vi "WAV_Master.vi"() -> ()   [LabVIEW 2022 SP3]
uses:
  PreferencesControl.ctl
  <vilib>/Utility/miscctls.llb/LVSelectionTypeDef.ctl
  <vilib>/Utility/error.llb/Trim Whitespace One-Sided.vi
panel:
  out "names":string[](array[string])
  out "wfm":waveform(dbl)[](graph)
  in  "Tab Control":enum32{"Intro", "Params", "Settings", "Saving"}(tab)
  out "Number of taps":i32
  out "raw file":string
  in  "Set Name":string="H"
  in  "Tap number":u32=1
  in  "Position":u32=1
  in  "Settings":T1={"Name of test"="name", "Date"=timestamp(0 s since 1904-01-01), "Location"="Home", "Template"="wav translator", "Soundcard"="OCTA-CAPTURE", "resolution"=32, "Sampling rate"=48000, "Ch1 Gain "=10.0, "Ch2 Gain"=20.0, "Sample time (s)"=0.3, "Pre-trigger (s)"=0.001, "Hammer Threshold"=0.01, "Positions"=12, "Taps/Position"=5, "Set Names"="H,V", "Freq resolution"=1.0, "Hammer cutoff"=0.025, "Mic cutoff"=0.25, "Double bounce "=0.01, "Hammer Cal"=23.6, "dB Offset"=0.0, "Accel Cal"=1.014, "Vibrometer Cal"=1.0, "Mic Cal"=48.5, "Output"=2, "Voltage Cal"=3.8, "Vibrometer Port"="ASRL27::INSTR", "Range"=50, "High Pass"=2, "Bandwidth"=25, "X Range"=[{"Minimum"=200.0, "Maximum"=10000.0, "Increment"=2500.0, "Minor Increment"=500.0, "Start"=2500.0}, {"Minimum"=0.0, "Maximum"=0.05, "Increment"=0.025, "Minor Increment"=0.0025, "Start"=0.0}, {"Minimum"=0.0, "Maximum"=0.3, "Increment"=0.1, "Minor Increment"=0.01, "Start"=0.0}, {"Minimum"=200.0, "Maximum"=10000.0, "Increment"=10.0, "Minor Increment"=100.0, "Start"=1000.0}], "Y Range"=[{"Minimum"=-25.0, "Maximum"=0.0, "Increment"=5.0, "Minor Increment"=1.0, "Start"=-25.0}, {"Minimum"=-0.1, "Maximum"=1.0, "Increment"=0.25, "Minor Increment"=0.05, "Start"=0.0}, {"Minimum"=-1.0, "Maximum"=1.0, "Increment"=0.5, "Minor Increment"=0.1, "Start"=-1.0}, {"Minimum"=-10.0, "Maximum"=30.0, "Increment"=10.0, "Minor Increment"=0.5, "Start"=-10.0}], "dB Spread"=40.0, "Trigger"=0, "Ch_1"=2, "Ch_2"=1, "flip?"=FALSE, "60Hz"=FALSE, "Time offset"=0.0, "Piezo Cal"=1.0, "Default Notes"=""} {"Ch_2" min=1 step=1; "Ch_1" min=1 max=100 step=1; "Trigger" items=["Hammer (force)", "Self-tap", "Spacebar"]; "Bandwidth" items=["1 kHz"=1, "5 kHz"=5, "10 kHz"=10, "25 kHz"=25, "50 kHz"=50, "100 kHz"=100]; "High Pass" items=["Off", "13 Hz", "104 Hz"]; "Range" items=["10 mm/s"=1, "20 mm/s"=2, "50 mm/s"=5, "100 mm/s"=10, "200 mm/s"=20, "500 mm/s"=50, "1 m/s"=100, "2 m/s"=200]; "Output" items=["Accelerometer", "Speed (from acceleration)", "Microphone", "Vibrometer", "Piezo"]; "Voltage Cal" format="%#_13g"; "Ch2 Gain" format="%#_13g"; "Ch1 Gain" format="%#_13g"; "Double bounce" min=0.0; "Mic cutoff" min=0.0 format="%#_4g"; "Hammer cutoff" min=0.0 format="%#_4g"; "Freq resolution" min=0.0; "Pre-trigger (s)" format="%#_13g"; "Date" format="%<%H:%M\n%d/%m/%y>T"; "resolution" items=["16 bit"=16, "24 bit"=24, "32 bit"=32]; "Sampling rate" items=["22050 samp/s"=22050, "44100 samp/s"=44100, "48000 samp/s"=48000]}
  in  "Test Name":string
  in  "Files":i32(listbox)=-1
  in  "Save Button":bool
  in  "Instrument Name":string(combo)
  in  "View Settings":bool
  in  "wav folder path":path
  out "FRF":cluster{"x0":dbl, "df":dbl, dbl[]}(graph)
  in  "play selection":bool
  out "File name":string
  out "data":T2={"Hammer"=[], "Hammer Spectra"=[{1.0, "df"=1.0, "FFT {X}"=array[24000 elements]}], "Microphone"=[{0.0, "dt"=2.0833333333333333e-05, "Y"=array[14400 elements]}], "Microphone Spectra"=[{"x0"=1.0, "df"=1.0, array[24000 elements]}], "Average FRF"=[{1.0, "df"=1.0, array[24000 elements]}, {1.0, "df"=1.0, array[24000 elements]}]}
  in  "Back":bool
  out "Slide":u8(slide) scale=0.0..100.0
  # "Welcome To The WAV File Translator"
  # "This will translate a wav file and let you play it"
  # "1. Select a folder of wav files\nHit the folder button or drag a file on"
  # "2. Define an instrument and settings\nAdd to an existing or create a new instrument\nand edit settings (or use defaults)"
  # "3. Translate the data\nMake sure the data looks good"
  # "4. Specify start Set, position, and hit\nall gets added to the data file name"
  # "5. Repeat or Close\nSelect a new file or close the window"
  # "Hz"
  # "dB"
  # "dB"
  # "sec"
  # "sec"
  # "mV/Pa"
  # "mV/m/s2"
  # "mV/mm/s"
  # "V/N"
  # "sec"
  # "sec"
  # "mV/N"
  # "a.u."
  # "a.u."
  # "sec"
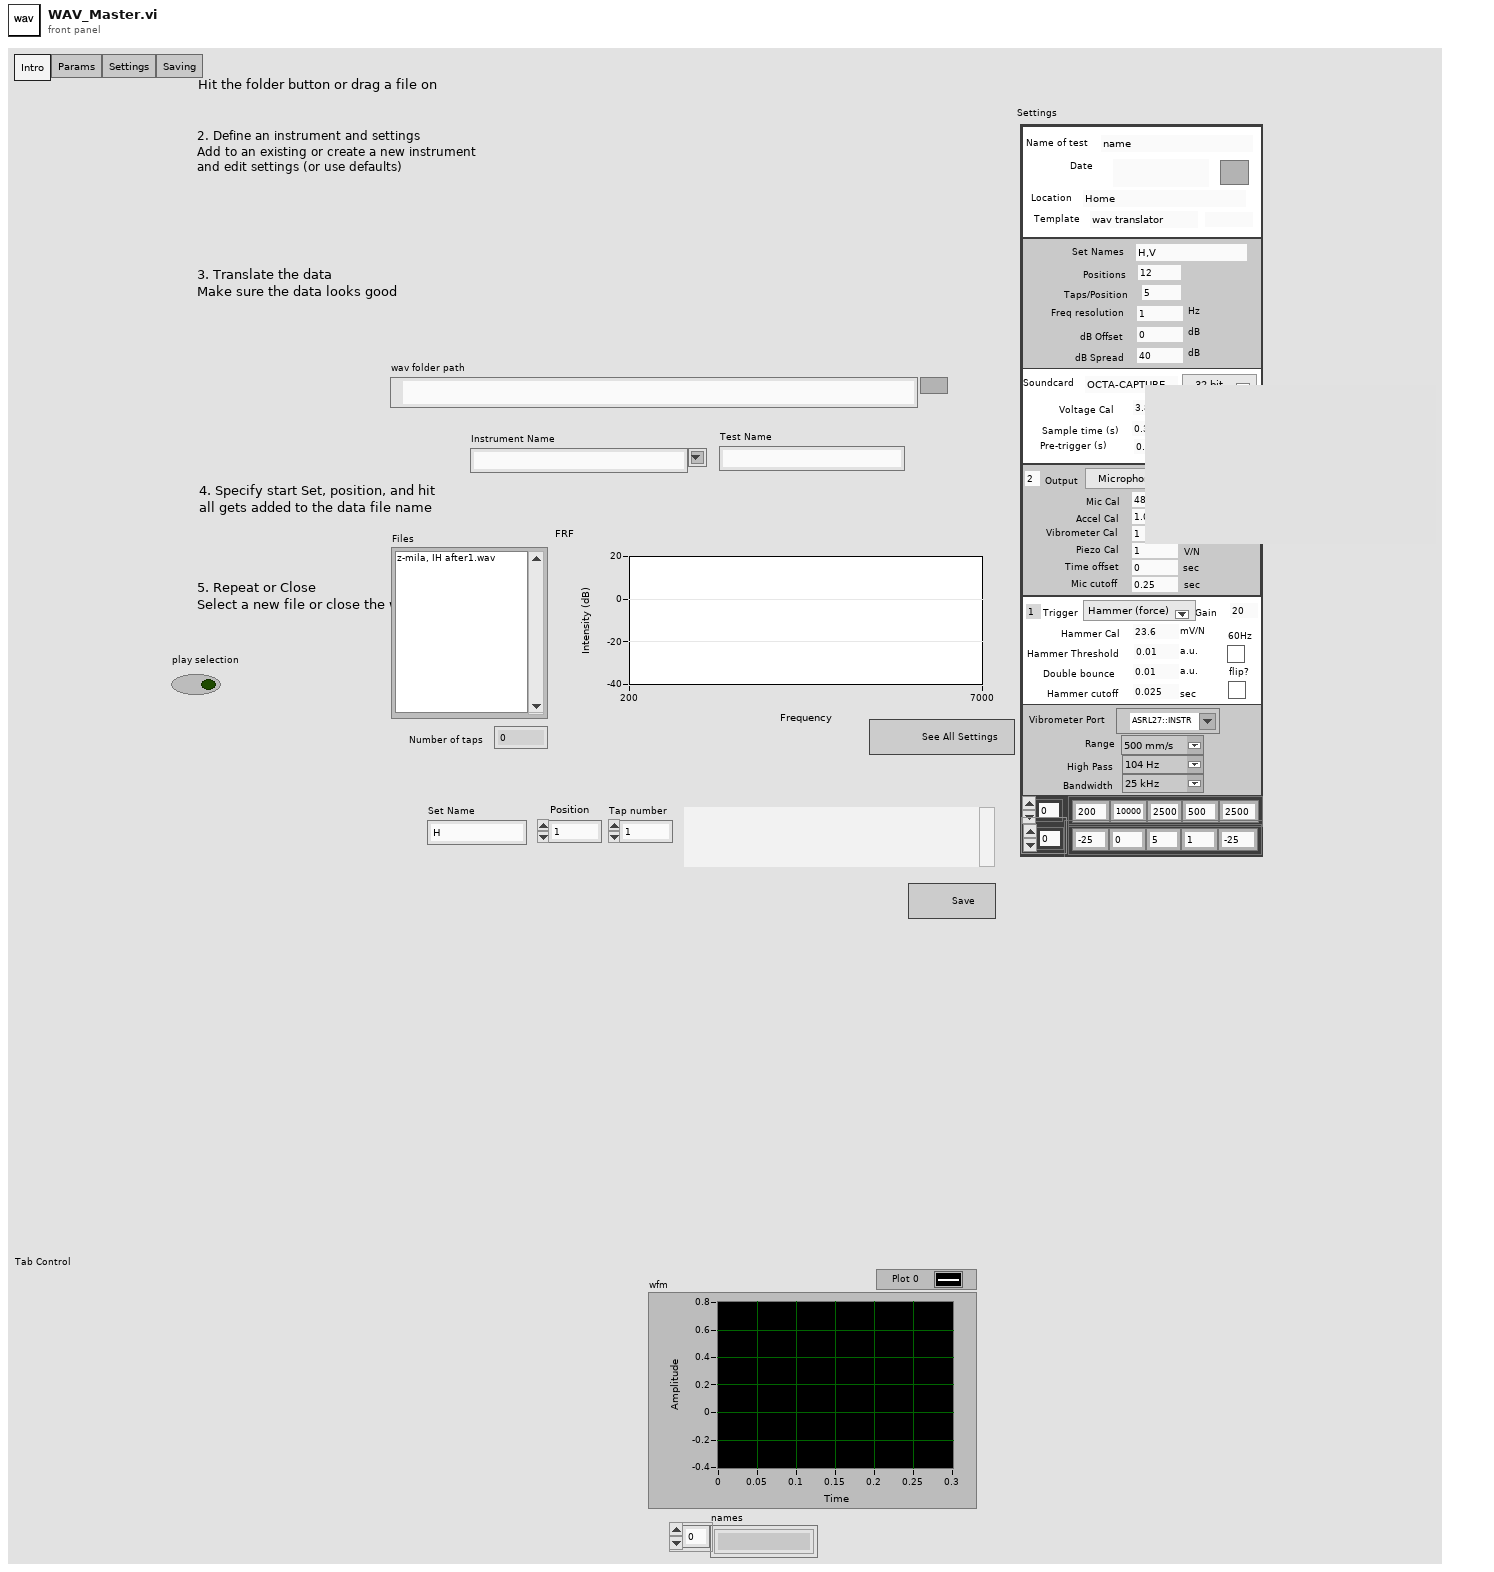
[diagram p1: front panel]
types:
  T1 = typedef "PreferencesControl.ctl" = cluster{"Name of test":string, "Date":timestamp, "Location":string, "Template":string, "Soundcard":string, "resolution":u16, "Sampling rate":u16, "Ch1 Gain ":dbl, "Ch2 Gain":dbl, "Sample time (s)":dbl, "Pre-trigger (s)":dbl, "Hammer Threshold":dbl, "Positions":i16, "Taps/Position":i16, "Set Names":string, "Freq resolution":dbl, "Hammer cutoff":dbl, "Mic cutoff":dbl, "Double bounce ":dbl, "Hammer Cal":dbl, "dB Offset":dbl, "Accel Cal":dbl, "Vibrometer Cal":dbl, "Mic Cal":dbl, "Output":u16, "Voltage Cal":dbl, "Vibrometer Port":refnum<visa-resource-name>, "Range":u16, "High Pass":u16, "Bandwidth":u16, "X Range":cluster{"Minimum":dbl, "Maximum":dbl, "Increment":dbl, "Minor Increment":dbl, "Start":dbl}[], "Y Range":cluster{"Minimum":dbl, "Maximum":dbl, "Increment":dbl, "Minor Increment":dbl, "Start":dbl}[], "dB Spread":dbl, "Trigger":u16, "Ch_1":u8, "Ch_2":u8, "flip?":bool, "60Hz":bool, "Time offset":dbl, "Piezo Cal":dbl, "Default Notes":string}
  T2 = cluster{"Hammer":cluster{dbl, "dt":dbl, "Y":dbl[]}[], "Hammer Spectra":cluster{dbl, "df":dbl, "FFT {X}":dbl[]}[], "Microphone":cluster{dbl, "dt":dbl, "Y":dbl[]}[], "Microphone Spectra":cluster{"x0":dbl, "df":dbl, dbl[]}[], "Average FRF":cluster{dbl, "df":dbl, dbl[]}[]}
  T3 = enum8{"Enabled", "Disabled", "Disabled and Grayed Out"}
  T4 = typedef "LVSelectionTypeDef.ctl" = cluster{"Selection Start":u32, "Selection End":u32}
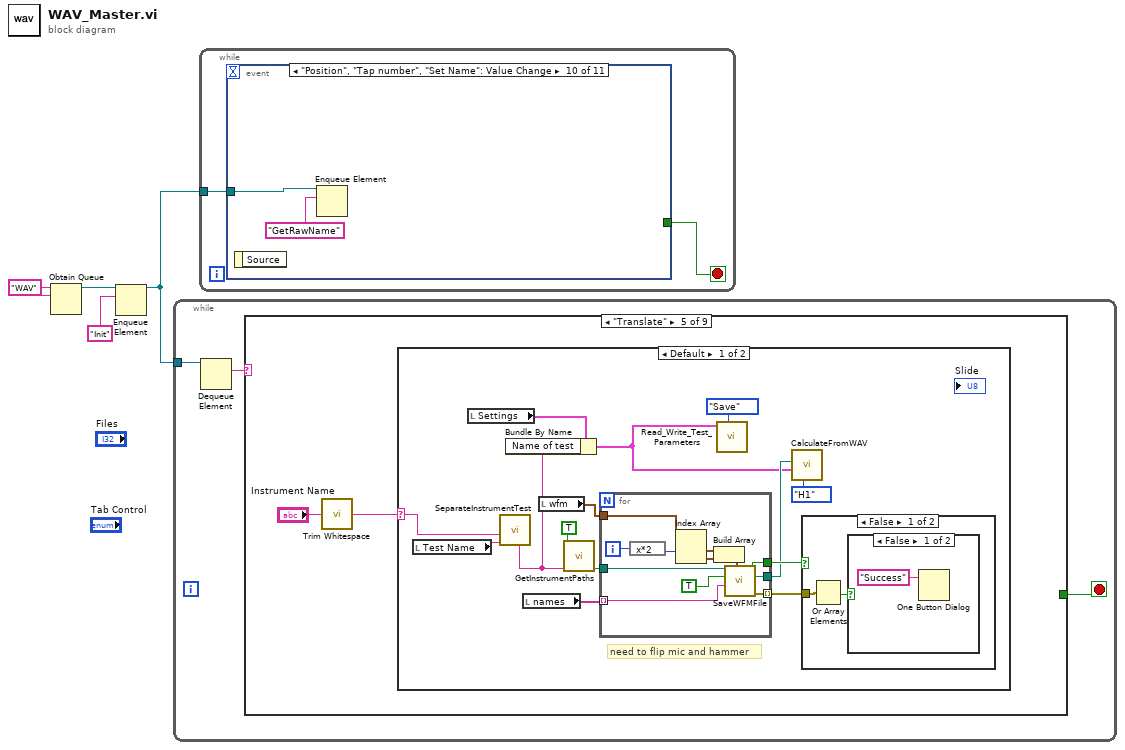
[diagram p0: block diagram]
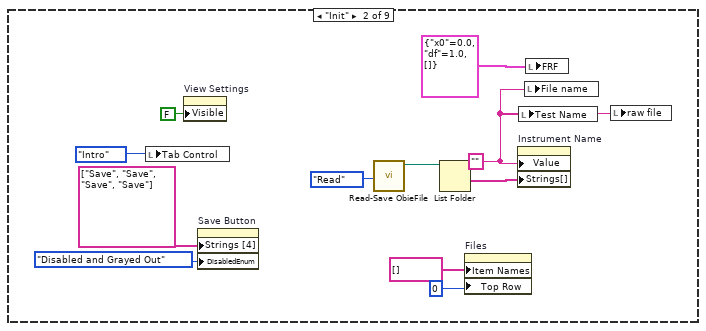
[diagram p3: hidden frame]
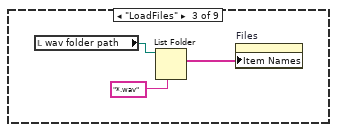
[diagram p4: hidden frame]
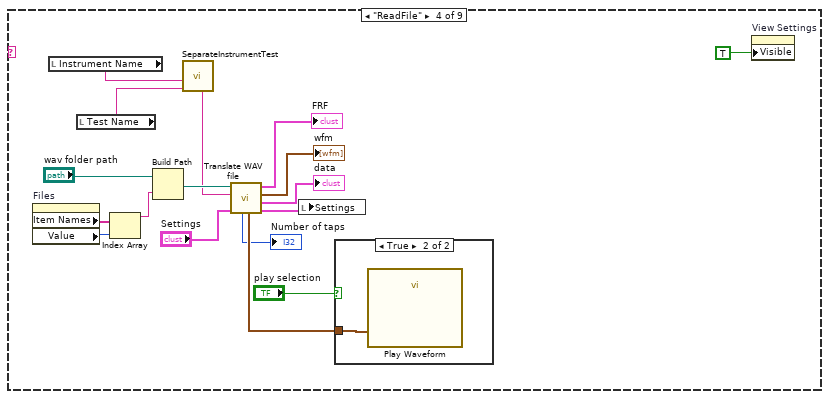
[diagram p5: hidden frame]
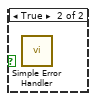
[diagram p7: hidden frame]
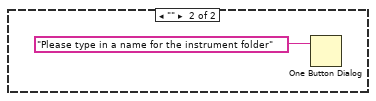
[diagram p9: hidden frame]
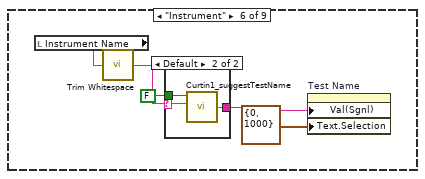
[diagram p10: hidden frame]
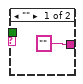
[diagram p11: hidden frame]
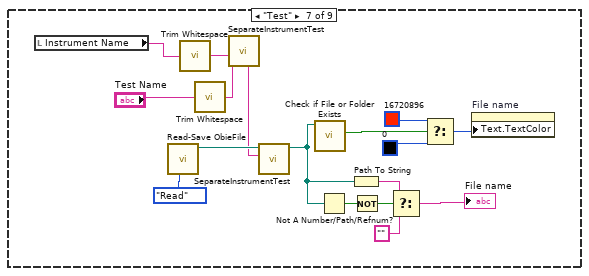
[diagram p12: hidden frame]
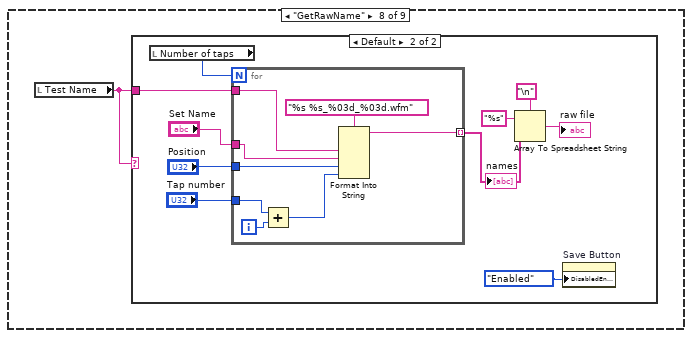
[diagram p13: hidden frame]
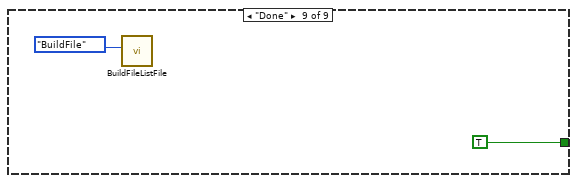
[diagram p15: hidden frame]
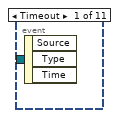
[diagram p16: hidden frame]
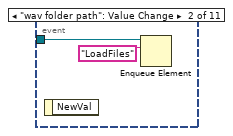
[diagram p17: hidden frame]
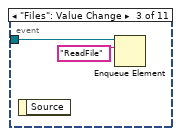
[diagram p18: hidden frame]
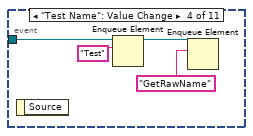
[diagram p19: hidden frame]
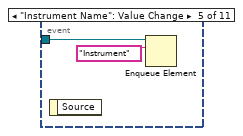
[diagram p20: hidden frame]
diagram:
  w4 = "WAV" ("name (unnamed)")
  n1 = Obtain Queue(name (unnamed)=w4, element data type=w4) -> (queue out=w2:refnum<queue>)  [unwired: 3 in, 2 out]
  n2 = Enqueue Element(queue=w2, element="Init") -> (queue out=w1:refnum<queue>)  [unwired: 2 in, 2 out]
  n3 = while {
    tunnel: w1 -> [w7]
    stop <- w5 stop-if-true
    n4 = Dequeue Element(queue=w7) -> (element=w6:string)  [unwired: 2 in, 3 out]
    n5 = case shown="\"Translate\"" w6 {
      tunnel: [_ _ _ _ _ _ _ _ TRUE ("Discard?")] -> w5
      frame Default {
      }
      frame "Init" {
        w8 = "" ("Value (Signaling)")
        n6 = local write "Tab Control"(enum32{"Intro", "Params", "Settings"}."Intro" ("Tab Control")) -> ()
        n7 = property on="View Settings" class="Bool"("Visible"=FALSE) -> ()  [unwired: 2 in, 2 out]
        n8 = property on="Save Button" class="Bool"("Strings [4]"=string[] ["Save", "Save", "Save", "Save"], "DisabledEnum"=T3."Disabled and Grayed Out" ("Disabled")) -> ()  [unwired: 2 in, 2 out]
        n9 = call "Read-Save ObieFile.vi"("Task"=enum16{"Save", "Read"}."Read") -> ("DataPath Out"=w15:path)  [unwired: 8 in, 2 out]
        n10 = List Folder(path=w15) -> (folder names=w14:string[])  [unwired: 3 in, 3 out]
        n11 = property on="Files" class="LstBox (strict)"("Item Names"=string[] [], "Top Row"=0) -> ()  [unwired: 2 in, 2 out]
        n12 = property on="Instrument Name" class="CmbBox"("Value"=w8, "Strings[]"=w14) -> ()  [unwired: 2 in, 2 out]
        n13 = local write "Test Name"(w8) -> ()
        n14 = local write "File name"(w8) -> ()
        n15 = local write "FRF"(cluster{"x0":dbl, "df":dbl, dbl[]} {"x0"=0.0, "df"=1.0, []} ("FRF")) -> ()
        n16 = local write "raw file"(w8) -> ()
      }
      frame "LoadFiles" {
        n17 = local read "wav folder path"() -> (w21:path)
        n18 = List Folder(path=w21, pattern="*.wav") -> (filenames=w19:string[])  [unwired: 2 in, 3 out]
        n19 = property on="Files" class="LstBox (strict)"("Item Names"=w19) -> ()  [unwired: 2 in, 2 out]
      }
      frame "ReadFile" {
        n20 = property on="Files" class="LstBox (strict)"() -> ("Item Names"=w33:string[], "Value"=w34:i32)  [unwired: 2 in, 2 out]
        n21 = local read "Instrument Name"() -> (w24:string)
        n22 = local read "Test Name"() -> (w25:string)
        n23 = Index Array(array=w33, index=w34) -> (element=w32:string)
        n24 = Build Path(base path="wav folder path", name or relative path=w32) -> (appended path=w30:path)
        n25 = call "SeparateInstrumentTest.vi"("test in"=w25, "Instrument in"=w24) -> ("Instrument -- test out"=w23:string)  [unwired: 5 in, 4 out]
        n26 = call "Translate WAV file.vi"("Settings"="Settings", "Name of test"=w23, "appended path"=w30) -> ("Settings Out"=w28:T1, 1:"data"=→"data":T2, "data 2"=→"wfm":waveform(dbl)[], "Average FRF out"=→"FRF":cluster{"x0":dbl, "df":dbl, dbl[]}, 4:"data"=w35:waveform(dbl)[], "# pts"=→"Number of taps":i32)  [unwired: 2 in, 1 out]
        n27 = local write "Settings"(w28) -> ()
        n28 = case shown="True" "play selection" {
          tunnel: w35 -> [_ w39]
          frame False {
          }
          frame True {
            n29 = call "Play Waveform"("Data"=w39) -> ()  [unwired: 18 in, 1 out]
          }
        }
        n30 = property on="View Settings" class="Bool"("Visible"=TRUE) -> ()  [unwired: 2 in, 2 out]
      }
      frame "Translate" {
        n31 = call <vilib>:"Trim Whitespace.vi"("string"="Instrument Name") -> ("trimmed string"=w40:string)  [unwired: 1 in]
        n32 = case shown="Default" w40 {
          selector: w40 -> [w50 _]
          frame Default {
            # "need to flip mic and hammer"
            n33 = local read "Test Name"() -> (w54:string)
            n34 = local read "Settings"() -> (w43:T1)
            n35 = call "SeparateInstrumentTest.vi"("test in"=w54, "Instrument in"=w50) -> ("Instrument -- test out"=w44:string)  [unwired: 5 in, 4 out]
            n36 = Bundle By Name(cluster=w43, "Name of test"=w44) -> (w42:T1)
            n37 = local read "names"() -> (w53:string[])
            n38 = local read "wfm"() -> (w46:waveform(dbl)[])
            n39 = call "GetInstrumentPaths.vi"("Instrument"=w44, "Build?"=TRUE) -> ("Path To Raw Folder"=w47:path)  [unwired: 5 in, 4 out]
            n40 = for {
              tunnel: w53 -> [w66] mode=indexing
              tunnel: [w65] -> w52 mode=indexing
              tunnel: [w64] -> w49
              tunnel: [w63] -> w48
              tunnel: w47 -> [w62]
              tunnel: w46 -> [w58]
              i -> [w57]
              n41 = expression code="x*2"(w57) -> (w56:i32)
              n42 = Index Array(array=w58, index #1=w56) -> (element #1=w61:waveform(dbl), element #2=w59:waveform(dbl))  [unwired: 1 in]
              n43 = Build Array(w61, w59) -> (w60:waveform(dbl)[])
              n44 = call "SaveWFMFile.vi"("Data"=w60, "New File"=w66, "Good point?"=TRUE, "Path To Raw Folder"=w62) -> ("error out"=w65:errorcluster, "new file path"=w63:path, "Canceled"=w64:bool)  [unwired: 4 in, 1 out]
            }
            n45 = call "Read_Write_Test_Parameters.vi"("Task"=enum16{"Save", "Read", "Clear"}."Save", "Settings"=w42) -> ()  [unwired: 8 in, 2 out]
            n46 = call "CalculateFromWAV.vi"("Method"=enum16{"Sqrt(H1H2)", "H1", "H2"}."H1", "Settings"=w42, "path"=w48) -> ()  [unwired: 4 in, 5 out]
            n47 = case shown="False" w49 {
              tunnel: w52 -> [w69 _]
              frame False {
                n48 = Or Array Elements(Boolean array=w69) -> (logical OR=w68:bool)
                n49 = case shown="False" w68 {
                  frame False {
                    n50 = One Button Dialog(message="Success") -> ()  [unwired: 1 in, 1 out]
                  }
                  frame True {
                    n51 = call <vilib>:"Simple Error Handler.vi"() -> ()  [unwired: 5 in, 5 out]
                  }
                }
              }
              frame True {
              }
            }
          }
          frame "" {
            n52 = One Button Dialog(message="Please type in a name for the instrument folder") -> ()  [unwired: 1 in, 1 out]
          }
        }
      }
      frame "Instrument" {
        n53 = local read "Instrument Name"() -> (w74:string)
        n54 = call <vilib>:"Trim Whitespace.vi"("string"=w74) -> ("trimmed string"=w73:string)  [unwired: 1 in]
        n55 = case shown="Default" w73 {
          selector: w73 -> [_ w80]
          tunnel: ["" w79] -> w76
          tunnel: FALSE ("Build?") -> [_ w78]
          frame "" {
          }
          frame Default {
            n56 = call "Curtin1_suggestTestName.vi"("instrument"=w80, "Build?"=w78) -> ("Suggested Test"=w79:string)  [unwired: 9 in]
          }
        }
        n57 = property on="Test Name" class="Str"("Val(Sgnl)"=w76, "Text.Selection"=T4 {"Selection Start"=0, "Selection End"=1000}) -> ()  [unwired: 2 in, 2 out]
      }
      frame "Test" {
        n58 = local read "Instrument Name"() -> (w81:string)
        n59 = call "Read-Save ObieFile.vi"("Task"=enum16{"Save", "Read"}."Read") -> ("DataPath Out"=w87:path)  [unwired: 8 in, 2 out]
        n60 = call <vilib>:"Trim Whitespace.vi"("string"=w81) -> ("trimmed string"=w84:string)  [unwired: 1 in]
        n61 = call <vilib>:"Trim Whitespace.vi"("string"="Test Name") -> ("trimmed string"=w83:string)  [unwired: 1 in]
        n62 = call "SeparateInstrumentTest.vi"("test in"=w83, "Instrument in"=w84) -> ("Instrument -- test out"=w85:string)  [unwired: 5 in, 4 out]
        n63 = call "SeparateInstrumentTest.vi"("Instrument"=w85, "path in"=w87) -> ("path out"=w86:path)  [unwired: 5 in, 4 out]
        n64 = call <vilib>:"Check if File or Folder Exists.vi"("path"=w86) -> ("file or folder exists?"=w89:bool)  [unwired: 8 in, 2 out]
        n65 = Not A Number/Path/Refnum?(number/path/refnum=w86) -> (NaN/Path/Refnum?=w97:bool)
        n66 = Path To String(path=w86) -> (string=w96:string)
        n67 = Not(x=w97) -> (.not. x?=w95:bool)
        n68 = Select(t=w96, s=w95, f="") -> (s? t:f=→"File name":string)
        n69 = Select(t=u32 16720896, s=w89, f=u32 0) -> (s? t:f=w94:u32)
        n70 = property on="File name" class="Str"("Text.TextColor"=w94) -> ()  [unwired: 2 in, 2 out]
      }
      frame "GetRawName" {
        n71 = local read "Test Name"() -> (w98:string)
        n72 = case shown="Default" w98 {
          tunnel: w98 -> [_ w105]
          frame "" {
          }
          frame Default {
            n73 = local read "Number of taps"() -> (w103:i32)
            n74 = for {
              N: w103 -> [_]
              tunnel: "Tap number" -> [w111]
              tunnel: "Position" -> [w116]
              tunnel: w105 -> [w114]
              tunnel: "Set Name" -> [w113]
              tunnel: [w109] -> w102 mode=indexing
              i -> [w112]
              n75 = Add(x=w111, y=w112) -> (x+y=w110:u32)
              n76 = Format Into String(format string="%s %s_%03d_%03d.wfm", w114, w113, w116, w110) -> (resulting string=w109:string)  [unwired: 2 in, 1 out]
            }
            "names" <- w102
            n77 = Array To Spreadsheet String(delimiter (Tab)="\n", array=w102, 3:"%s" ("format string")) -> (spreadsheet string=→"raw file":string)
            n78 = property on="Save Button" class="Bool"("DisabledEnum"=T3."Enabled" ("Disabled")) -> ()  [unwired: 2 in, 2 out]
          }
        }
      }
      frame "Done" {
        n79 = call "BuildFileListFile.vi"("Task"=enum16{"BuildFile", "ReadFile"}."BuildFile") -> ()  [unwired: 9 in, 2 out]
      }
    }
  }
  n80 = while {
    tunnel: w1 -> [w120]
    stop <- w119 stop-if-true
    n81 = event shown="[9] \"Position\", \"Tap number\", \"Set Name\": Value Change" {
      selector: _ -> [_ _ _ _ _ _ _ _ _ _ _]
      dyn-events: _ -> [_ _ _ _ _ _ _ _ _ _ _]
      timeout: _ -> [_ _ _ _ _ _ _ _ _ _ _]
      tunnel: w120 -> [_ w122 w124 w128 w130 w132 w134 _ _ w137 w139]
      tunnel: [_ _ _ _ _ _ _ _ _ _ w141] -> w119
      event Timeout {
        n82 = event-data() -> ()  [unwired: 1 in, 3 out]
      }
      event "wav folder path": Value Change {
        n83 = event-data() -> ()  [unwired: 1 in, 1 out]
        n84 = Enqueue Element(queue=w122, element="LoadFiles") -> ()  [unwired: 2 in, 3 out]
      }
      event "Files": Value Change {
        n85 = event-data() -> ()  [unwired: 1 in, 1 out]
        n86 = Enqueue Element(queue=w124, element="ReadFile") -> ()  [unwired: 2 in, 3 out]
      }
      event "Test Name": Value Change {
        n87 = event-data() -> ()  [unwired: 1 in, 1 out]
        n88 = Enqueue Element(queue=w128, element="Test") -> (queue out=w125:refnum<queue>)  [unwired: 2 in, 2 out]
        n89 = Enqueue Element(queue=w125, element="GetRawName") -> ()  [unwired: 2 in, 3 out]
      }
      event "Instrument Name": Value Change {
        n90 = event-data() -> ()  [unwired: 1 in, 1 out]
        n91 = Enqueue Element(queue=w130, element="Instrument") -> ()  [unwired: 2 in, 3 out]
      }
      event "play selection": Value Change {
        n92 = event-data() -> ()  [unwired: 1 in, 1 out]
        n93 = Enqueue Element(queue=w132, element="ReadFile") -> ()  [unwired: 2 in, 3 out]
      }
      event "Save Button": Value Change {
        n94 = event-data() -> ()  [unwired: 1 in, 1 out]
        n95 = Enqueue Element(queue=w134, element="Translate") -> ()  [unwired: 2 in, 3 out]
      }
      event "Back": Value Change {
        n96 = event-data() -> ()  [unwired: 1 in, 1 out]
        n97 = local write "Tab Control"(enum32{"Intro", "Params", "Settings"}."Intro" ("Tab Control")) -> ()
      }
      event "View Settings": Value Change {
        n98 = event-data() -> ()  [unwired: 1 in, 1 out]
        n99 = local write "Tab Control"(enum32{"Intro", "Params", "Settings"}."Params" ("Tab Control")) -> ()
      }
      event "Position", "Tap number", "Set Name": Value Change {
        n100 = event-data() -> ()  [unwired: 1 in, 1 out]
        n101 = Enqueue Element(queue=w137, element="GetRawName") -> ()  [unwired: 2 in, 3 out]
      }
      event Panel Close? {
        w141 = TRUE ("Discard?")
        n102 = event-data() -> ()  [unwired: 1 in, 1 out]
        n103 = Enqueue Element(queue=w139, element="Done") -> ()  [unwired: 2 in, 3 out]
        n104 = event-data("Discard?"=w141) -> ()  [unwired: 1 in, 1 out]
      }
    }
  }
